vi "AssetInterface_Read Process Name.vi"(11 "Grid in":refnum<class "Grid.lvclass">) -> (2 "Process Name":string, 3 "Grid out":refnum<class "Grid.lvclass">)   [LabVIEW 2015, in "Grid.lvclass"]
uses:
  Grid.lvclass
  Grid.lvclass/Grid.ctl
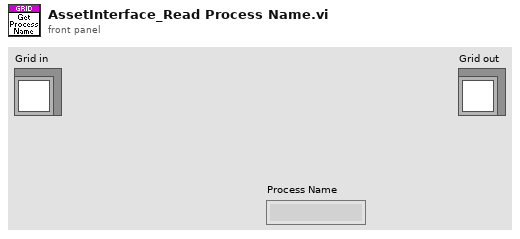
[diagram p1: front panel]
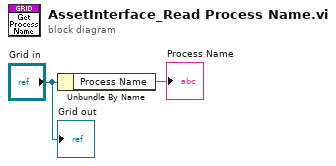
[diagram p0: block diagram]
diagram:
  n1 = Unbundle By Name("Grid in") -> ("Process Name"=→"Process Name":string)
  "Grid out" <- "Grid in"
